vi "Get Object.vi"(6 "Version ID":string, 8 "error in (no error)":errorcluster, 9 "Request Parameters":T2, 10 "Object Key":string, 11 "Bucket in":refnum<class "Bucket.lvclass">) -> (0 "error out":errorcluster, 1 "Results":T1, 2 "Data":string, 3 "Bucket out":refnum<class "Bucket.lvclass">)   [LabVIEW 2015, in "NI_AWS_S3.lvlib" / "Bucket.lvclass"]
uses:
  Bucket.lvclass
  GET Object Request Parameters.ctl
  Core/Request Range.ctl
  GET Object Result Parameters.ctl
  Core/HTTP Request/Request Options.ctl
  Core/HTTP Request/Name Value Pair.ctl
  Core/HTTP Request/Region handling.ctl
  Core/HTTP Request/URL formatting.ctl
  Bucket.lvclass/Bucket.ctl
  Read Name.vi
  Core/HTTP Request/HTTP Request.lvclass
  Object/Object.lvlib
  NI_AWS_S3.lvlib
  Core/NI_AWS_Core.lvlib
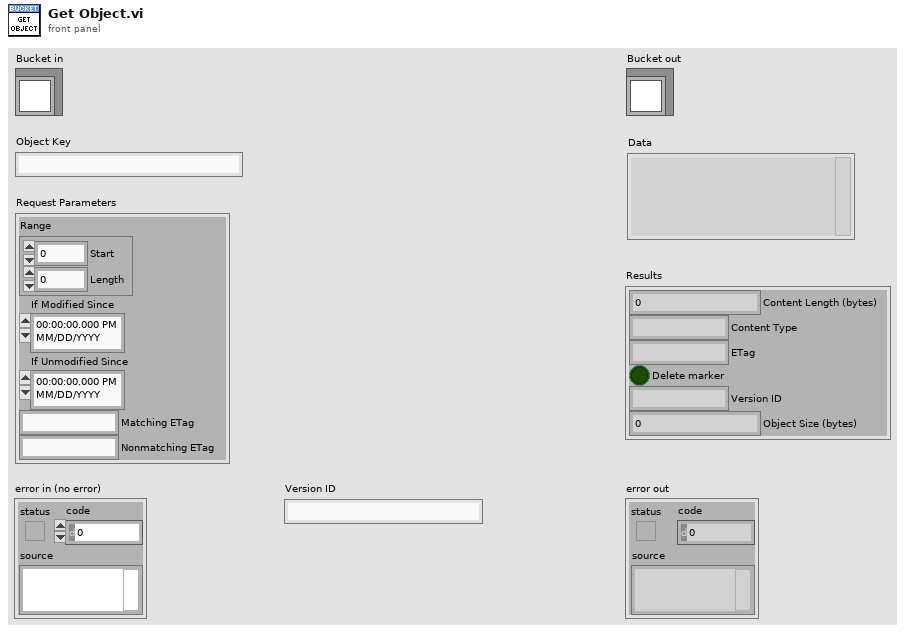
[diagram p1: front panel]
types:
  T1 = typedef "NI_AWS_S3.lvlib/GET Object Result Parameters.ctl" = cluster{"Content Length (bytes)":u64, "Content Type":string, "ETag":string, "Delete marker":bool, "Version ID":string, "Object Size (bytes)":u64}
  T2 = typedef "NI_AWS_S3.lvlib/GET Object Request Parameters.ctl" = cluster{"Range":T3, "If Modified Since":timestamp, "If Unmodified Since":timestamp, "Matching ETag":string, "Nonmatching ETag":string}
  T3 = typedef "NI_AWS_Core.lvlib/Request Range.ctl" = cluster{"Start":i64, "Length":i64}
  T4 = typedef "NI_AWS_Core.lvlib/HTTP Request.lvclass/Region handling.ctl" = enum16{"use region everywhere", "use region (authentication only)", "use region (URL only)", "ignore region everwhere"}
  T5 = typedef "NI_AWS_Core.lvlib/HTTP Request.lvclass/Request Options.ctl" = cluster{"request headers":T6[], "request parameters":T6[], "request body":string, "region handling":T4, "URL formatting":T7}
  T6 = typedef "NI_AWS_Core.lvlib/HTTP Request.lvclass/Name Value Pair.ctl" = cluster{"name":string, "value":string}
  T7 = typedef "NI_AWS_Core.lvlib/HTTP Request.lvclass/URL formatting.ctl" = enum16{"region-", "region."}
  T8 = typedef "NI_AWS_Core.lvlib/HTTP Request.lvclass/Response.ctl" = cluster{"Headers":string, "Body":string}
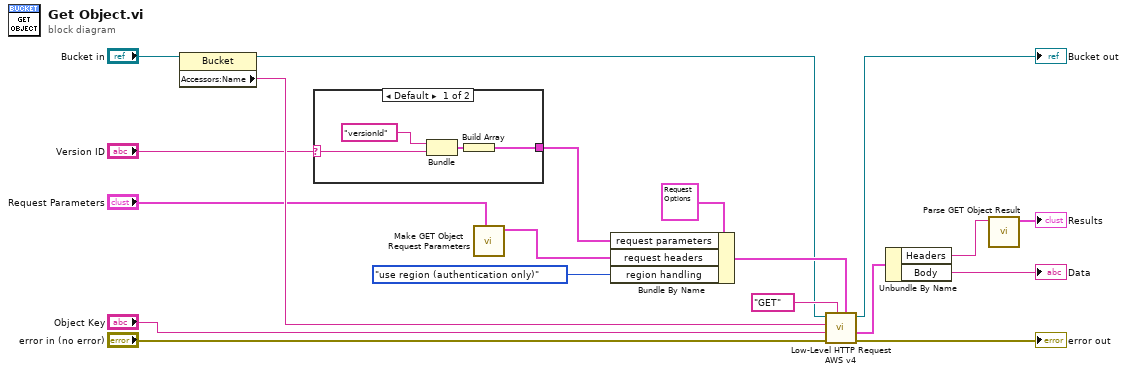
[diagram p0: block diagram]
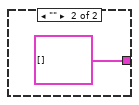
[diagram p2: hidden frame]
diagram:
  n1 = property class="Bucket"(reference="Bucket in") -> (reference out=w1:refnum<class "Bucket.lvclass">, "Accessors:Name"=w18:string)  [unwired: 1 in, 1 out]
  n2 = case shown="Default" "Version ID" {
    selector: "Version ID" -> [w20 _]
    tunnel: [w21 T6[] [] ("request parameters")] -> w12
    frame Default {
      n3 = Bundle("versionId", w20) -> (w22:cluster{string, string})  [unwired: 1 in]
      n4 = Build Array(w22) -> (w21:cluster{string, string}[])
    }
    frame "" {
    }
  }
  n5 = call "Make GET Object Request Parameters.vi"("GET Object Request Parameters"="Request Parameters") -> ("HTTP Headers"=w9:T6[])  [unwired: 10 in]
  n6 = Bundle By Name(cluster=T5 {"request headers"=[], "request parameters"=[], "request body"="", "region handling"=enum."use region everywhere", "URL formatting"=enum."region."} ("Request Options"), "request parameters"=w12, "request headers"=w9, "region handling"=Region_handling."use region (authentication only)") -> (w3:T5)
  n7 = call "Low-Level HTTP Request AWS v4.vi"("Request Options"=w3, "HTTP-Verb"="GET", "error in (no error)"="error in (no error)", "URL Suffix"="Object Key", "URL Prefix"=w18, "AWS Core in"=w1) -> ("error out"=→"error out":errorcluster, "Response"=w5:T8, "AWS Core out"=→"Bucket out":refnum<class "Bucket.lvclass">)  [unwired: 2 in, 1 out]
  n8 = Unbundle By Name(w5) -> ("Headers"=w7:string, "Body"=→"Data":string)
  n9 = call "Parse GET Object Result.vi"("Response header"=w7) -> ("GetObjectResult"=→"Results":T1)  [unwired: 9 in, 1 out]
